vi "Expand.vi"(8 "error in (no error)":errorcluster, 10 "Expand Direction":enum16{"Height", "Width", "Both"}(ring)=enum."Both", 11 "Brick Wall in":refnum<class "Bricks.lvclass">) -> (0 "error out":errorcluster, 3 "Brick Wall out":refnum<class "Bricks.lvclass">)   [LabVIEW 2015, in "Bricks.lvclass"]
uses:
  Bricks.lvclass
  Bricks.lvclass/Bricks.ctl
  Type Defs/Direction Enum.ctl
  Common/Position.ctl
  Square/Board Size.vi
  SubVIs/Read-Only Globals.vi
  Common/Common.lvlib
  Type Defs/SB Type Defs.lvlib
  Square/Square.lvclass
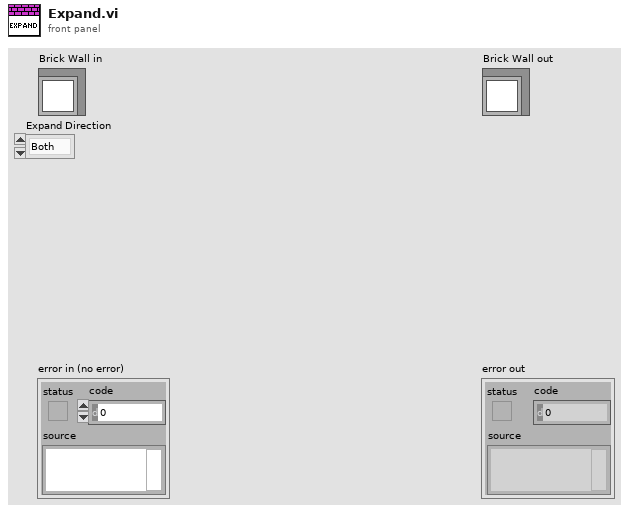
[diagram p1: front panel]
types:
  T1 = typedef "SB Type Defs.lvlib/Direction Enum.ctl" = enum16{"NW", "N", "NE", "E", "SE", "S", "SW", "W"}
  T2 = typedef "Common.lvlib/Position.ctl" = cluster{"Column":i32, "Row":i32}
  T3 = typedef "Bricks.lvclass/MasonLines.ctl" = cluster{"NMasonLine":i32, "EMasonLine":i32, "SMasonLine":i32, "WMasonLine":i32}
  T4 = typedef "Bricks.lvclass/SpawnLines.ctl" = cluster{"NSpawn":i32, "ESpawn":i32, "SSpawn":i32, "WSpawn":i32}
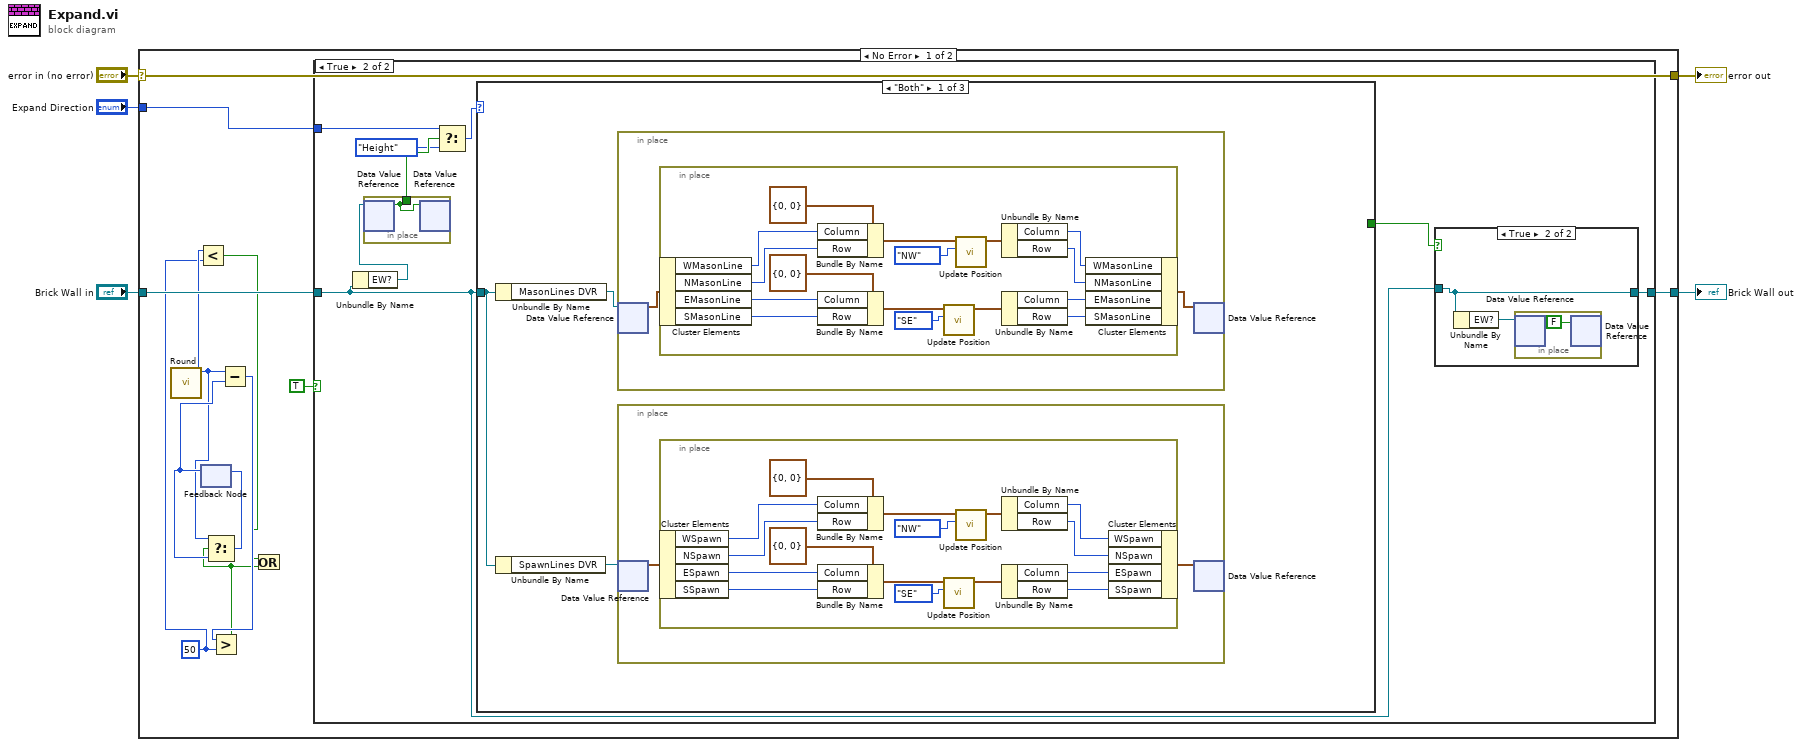
[diagram p0: block diagram]
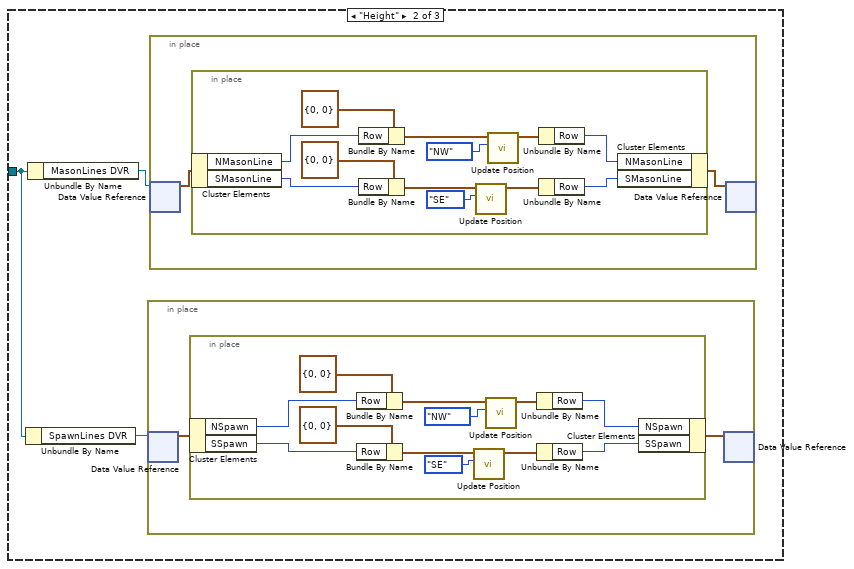
[diagram p4: hidden frame]
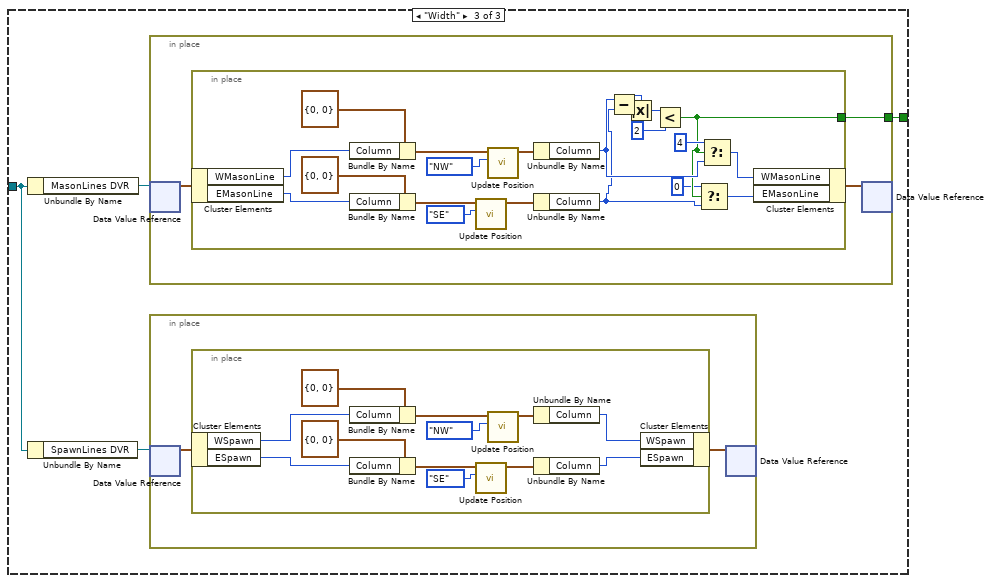
[diagram p5: hidden frame]
diagram:
  n1 = case shown="No Error" "error in (no error)" {
    selector: "error in (no error)" -> [w17 w144]
    tunnel: [w17 w144] -> w4
    tunnel: [w16 w143] -> w2
    tunnel: "Brick Wall in" -> [w15 w143]
    tunnel: "Expand Direction" -> [w14 _]
    frame No Error {
      w8 = 50 ("y")
      n2 = call "Round.vi"() -> ("Round"=w9:i32)  [unwired: 11 in]
      n3 = Less?(x=w9, y=w8) -> (x < y?=w7:bool)
      n4 = feedback #1() -> (w11:i32)  [unwired: 1 in]
      n5 = Subtract(x=w9, y=w11) -> (x-y=w12:i32)
      n6 = Greater?(x=w12, y=w8) -> (0:w10:bool)
      n7 = Select(t=w9, s=w10, f=w11) -> (s? t:f=w13:i32)
      n8 = feedback-in #1(w13) -> ()
      n9 = Or(x=w7, y=w10) -> ()  [unwired: 1 out]
      n10 = case shown="True" TRUE {
        tunnel: [w18 w26] -> w16
        tunnel: w15 -> [w18 w24]
        tunnel: w14 -> [_ w21]
        frame False {
        }
        frame True {
          n11 = Unbundle By Name(w24) -> ("EW?"=w23:refnum<data-value>)
          n12 = in-place {
            in-place-border: [w27] -> w22
            n13 = in-place-dvr #2(w23) -> (w27:bool)  [unwired: 1 out]
            n14 = in-place-dvr #2(w27) -> ()  [unwired: 2 out]
          }
          n15 = Select(t=w21, s=w22, f=enum16{"Height", "Width", "Both"}."Height") -> (s? t:f=w20:enum16{"Height", "Width", "Both"})
          n16 = case shown="\"Both\"" w20 {
            tunnel: w24 -> [w32 w71 w103]
            tunnel: [_ _ w102] -> w25
            frame "Both" {
              n17 = Unbundle By Name(w32) -> ("MasonLines DVR"=w34:refnum<data-value>)
              n18 = Unbundle By Name(w32) -> ("SpawnLines DVR"=w33:refnum<data-value>)
              n19 = in-place {
                n20 = in-place-dvr #3(w34) -> (w54:T3)  [unwired: 1 out]
                n21 = in-place {
                  n22 = in-place-cluster #4(w54) -> ("WMasonLine"=w67:i32, "NMasonLine"=w66:i32, "EMasonLine"=w59:i32, "SMasonLine"=w58:i32)
                  n23 = Bundle By Name(cluster=T2 {"Column"=0, "Row"=0} ("Position in"), "Column"=w67, "Row"=w66) -> (w68:T2)
                  n24 = Bundle By Name(cluster=T2 {"Column"=0, "Row"=0} ("Position in"), "Column"=w59, "Row"=w58) -> (w64:T2)
                  n25 = call "Update Position.vi"("Direction"=Direction_Enum."SE", "Position in"=w64) -> ("Position out"=w57:T2)  [unwired: 9 in]
                  n26 = call "Update Position.vi"("Direction"=Direction_Enum."NW", "Position in"=w68) -> ("Position out"=w62:T2)  [unwired: 9 in]
                  n27 = Unbundle By Name(w62) -> ("Column"=w61:i32, "Row"=w60:i32)
                  n28 = Unbundle By Name(w57) -> ("Column"=w56:i32, "Row"=w55:i32)
                  n29 = in-place-cluster #4("WMasonLine"=w61, "NMasonLine"=w60, "EMasonLine"=w56, "SMasonLine"=w55) -> (w53:T3)
                }
                n30 = in-place-dvr #3(w53) -> ()  [unwired: 2 out]
              }
              n31 = in-place {
                n32 = in-place-dvr #5(w33) -> (w36:T4)  [unwired: 1 out]
                n33 = in-place {
                  n34 = in-place-cluster #6(w36) -> ("WSpawn"=w49:i32, "NSpawn"=w48:i32, "ESpawn"=w41:i32, "SSpawn"=w40:i32)
                  n35 = Bundle By Name(cluster=T2 {"Column"=0, "Row"=0} ("Position in"), "Column"=w49, "Row"=w48) -> (w50:T2)
                  n36 = Bundle By Name(cluster=T2 {"Column"=0, "Row"=0} ("Position in"), "Column"=w41, "Row"=w40) -> (w46:T2)
                  n37 = call "Update Position.vi"("Direction"=Direction_Enum."SE", "Position in"=w46) -> ("Position out"=w39:T2)  [unwired: 9 in]
                  n38 = call "Update Position.vi"("Direction"=Direction_Enum."NW", "Position in"=w50) -> ("Position out"=w44:T2)  [unwired: 9 in]
                  n39 = Unbundle By Name(w44) -> ("Column"=w43:i32, "Row"=w42:i32)
                  n40 = Unbundle By Name(w39) -> ("Column"=w38:i32, "Row"=w37:i32)
                  n41 = in-place-cluster #6("WSpawn"=w43, "NSpawn"=w42, "ESpawn"=w38, "SSpawn"=w37) -> (w35:T4)
                }
                n42 = in-place-dvr #5(w35) -> ()  [unwired: 2 out]
              }
            }
            frame "Height" {
              n43 = Unbundle By Name(w71) -> ("SpawnLines DVR"=w72:refnum<data-value>)
              n44 = Unbundle By Name(w71) -> ("MasonLines DVR"=w73:refnum<data-value>)
              n45 = in-place {
                n46 = in-place-dvr #7(w72) -> (w75:T4)  [unwired: 1 out]
                n47 = in-place {
                  n48 = in-place-cluster #8(w75) -> ("NSpawn"=w84:i32, "SSpawn"=w78:i32)
                  n49 = Bundle By Name(cluster=T2 {"Column"=0, "Row"=0} ("Position in"), "Row"=w84) -> (w85:T2)
                  n50 = Bundle By Name(cluster=T2 {"Column"=0, "Row"=0} ("Position in"), "Row"=w78) -> (w82:T2)
                  n51 = call "Update Position.vi"("Direction"=Direction_Enum."SE", "Position in"=w82) -> ("Position out"=w77:T2)  [unwired: 9 in]
                  n52 = call "Update Position.vi"("Direction"=Direction_Enum."NW", "Position in"=w85) -> ("Position out"=w80:T2)  [unwired: 9 in]
                  n53 = Unbundle By Name(w80) -> ("Row"=w79:i32)
                  n54 = Unbundle By Name(w77) -> ("Row"=w76:i32)
                  n55 = in-place-cluster #8("NSpawn"=w79, "SSpawn"=w76) -> (w74:T4)
                }
                n56 = in-place-dvr #7(w74) -> ()  [unwired: 2 out]
              }
              n57 = in-place {
                n58 = in-place-dvr #9(w73) -> (w89:T3)  [unwired: 1 out]
                n59 = in-place {
                  n60 = in-place-cluster #10(w89) -> ("NMasonLine"=w98:i32, "SMasonLine"=w92:i32)
                  n61 = Bundle By Name(cluster=T2 {"Column"=0, "Row"=0} ("Position in"), "Row"=w98) -> (w99:T2)
                  n62 = Bundle By Name(cluster=T2 {"Column"=0, "Row"=0} ("Position in"), "Row"=w92) -> (w96:T2)
                  n63 = call "Update Position.vi"("Direction"=Direction_Enum."SE", "Position in"=w96) -> ("Position out"=w91:T2)  [unwired: 9 in]
                  n64 = call "Update Position.vi"("Direction"=Direction_Enum."NW", "Position in"=w99) -> ("Position out"=w94:T2)  [unwired: 9 in]
                  n65 = Unbundle By Name(w94) -> ("Row"=w93:i32)
                  n66 = Unbundle By Name(w91) -> ("Row"=w90:i32)
                  n67 = in-place-cluster #10("NMasonLine"=w93, "SMasonLine"=w90) -> (w88:T3)
                }
                n68 = in-place-dvr #9(w88) -> ()  [unwired: 2 out]
              }
            }
            frame "Width" {
              n69 = Unbundle By Name(w103) -> ("MasonLines DVR"=w105:refnum<data-value>)
              n70 = Unbundle By Name(w103) -> ("SpawnLines DVR"=w104:refnum<data-value>)
              n71 = in-place {
                in-place-border: [w120] -> w102
                n72 = in-place-dvr #11(w105) -> (w122:T3)  [unwired: 1 out]
                n73 = in-place {
                  in-place-border: [w126] -> w120
                  n74 = in-place-cluster #12(w122) -> ("WMasonLine"=w139:i32, "EMasonLine"=w134:i32)
                  n75 = Bundle By Name(cluster=T2 {"Column"=0, "Row"=0} ("Position in"), "Column"=w139) -> (w140:T2)
                  n76 = Bundle By Name(cluster=T2 {"Column"=0, "Row"=0} ("Position in"), "Column"=w134) -> (w137:T2)
                  n77 = call "Update Position.vi"("Direction"=Direction_Enum."SE", "Position in"=w137) -> ("Position out"=w133:T2)  [unwired: 9 in]
                  n78 = call "Update Position.vi"("Direction"=Direction_Enum."NW", "Position in"=w140) -> ("Position out"=w135:T2)  [unwired: 9 in]
                  n79 = Unbundle By Name(w135) -> ("Column"=w129:i32)
                  n80 = Unbundle By Name(w133) -> ("Column"=w125:i32)
                  n81 = Subtract(x=w129, y=w125) -> (x-y=w132:i32)
                  n82 = Absolute Value(x=w132) -> (abs(x)=w131:i32)
                  n83 = Less?(x=w131, y=2) -> (x < y?=w126:bool)
                  n84 = Select(t=0, s=w126, f=w125) -> (s? t:f=w124:i32)
                  n85 = Select(t=4, s=w126, f=w129) -> (s? t:f=w128:i32)
                  n86 = in-place-cluster #12("WMasonLine"=w128, "EMasonLine"=w124) -> (w121:T3)
                }
                n87 = in-place-dvr #11(w121) -> ()  [unwired: 2 out]
              }
              n88 = in-place {
                n89 = in-place-dvr #13(w104) -> (w107:T4)  [unwired: 1 out]
                n90 = in-place {
                  n91 = in-place-cluster #14(w107) -> ("WSpawn"=w116:i32, "ESpawn"=w110:i32)
                  n92 = Bundle By Name(cluster=T2 {"Column"=0, "Row"=0} ("Position in"), "Column"=w116) -> (w117:T2)
                  n93 = Bundle By Name(cluster=T2 {"Column"=0, "Row"=0} ("Position in"), "Column"=w110) -> (w114:T2)
                  n94 = call "Update Position.vi"("Direction"=Direction_Enum."SE", "Position in"=w114) -> ("Position out"=w109:T2)  [unwired: 9 in]
                  n95 = call "Update Position.vi"("Direction"=Direction_Enum."NW", "Position in"=w117) -> ("Position out"=w112:T2)  [unwired: 9 in]
                  n96 = Unbundle By Name(w112) -> ("Column"=w111:i32)
                  n97 = Unbundle By Name(w109) -> ("Column"=w108:i32)
                  n98 = in-place-cluster #14("WSpawn"=w111, "ESpawn"=w108) -> (w106:T4)
                }
                n99 = in-place-dvr #13(w106) -> ()  [unwired: 2 out]
              }
            }
          }
          n100 = case shown="True" w25 {
            tunnel: w24 -> [w28 w30]
            tunnel: [w28 w30] -> w26
            frame False {
            }
            frame True {
              n101 = Unbundle By Name(w30) -> ("EW?"=w29:refnum<data-value>)
              n102 = in-place {
                n103 = in-place-dvr #15(w29) -> ()  [unwired: 2 out]
                n104 = in-place-dvr #15(FALSE ("data value")) -> ()  [unwired: 2 out]
              }
            }
          }
        }
      }
    }
    frame Error {
    }
  }
  "error out" <- w4
  "Brick Wall out" <- w2
